vi "WriteData (Array of STR).vi"(6 "value index (0)":u64, 7 "Array of STR":string[](array[string]), 8 "error in (no error)":errorcluster, 9 "channel index (0)":u32, 10 "operation (0: create)":T2(ring)=enum."Create", 11 "Excel refnum":T1) -> (0 "error out":errorcluster, 3 "Excel refnum out":T1)   [LabVIEW 2020, in "NI_ExcelFile.lvlib"]
uses:
  <vilib>/express/express shared/NI_ExcelFile/NI_ExcelFile.lvlib
  <vilib>/express/express shared/NI_ExcelFile/Ctrls/ExcelRefnum.ctl
  <vilib>/express/express shared/NI_ExcelFile/Ctrls/MainData.ctl
  <vilib>/express/express shared/NI_ExcelFile/Ctrls/StreamMode.ctl
  <vilib>/express/express shared/NI_ExcelFile/Ctrls/TimeColumnMode.ctl
  <vilib>/express/express shared/NI_ExcelFile/Ctrls/FileAttribute.ctl
  <vilib>/express/express shared/NI_ExcelFile/Ctrls/Columns.ctl
  <vilib>/express/express shared/NI_ExcelFile/Ctrls/ColumnInfo.ctl
  <vilib>/express/express shared/NI_ExcelFile/Ctrls/DataType.ctl
  <vilib>/express/express shared/NI_ExcelFile/Ctrls/wd_recordInfo.ctl
  <vilib>/express/express shared/NI_ExcelFile/Ctrls/disk_TemplateFile.ctl
  <vilib>/express/express shared/NI_ExcelFile/Ctrls/meta_file.ctl
  <vilib>/express/express shared/NI_ExcelFile/Ctrls/meta_Block.ctl
  <vilib>/express/express shared/NI_ExcelFile/Ctrls/meta_BlockType.ctl
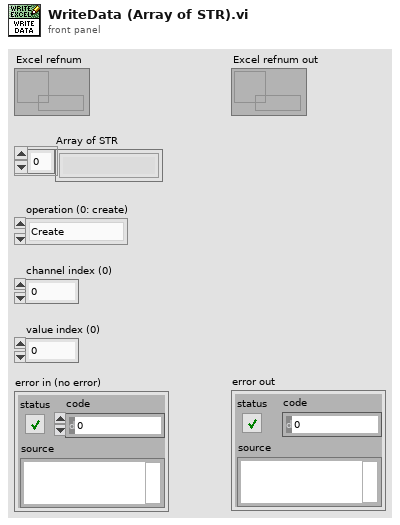
[diagram p1: front panel]
types:
  T1 = typedef "NI_ExcelFile.lvlib/ExcelRefnum.ctl" = refnum<data-value>
  T2 = enum16{"Append values", "Create", "Replace values at index", "Replace all values"}
  T3 = typedef "NI_ExcelFile.lvlib/DataType.ctl" = enum16{"DDT", "WFM", "Array of STR", "Array of DBL", "Array of I8", "Array of I16", "Array of I32", "Array of I64", "Array of SGL", "Array of U8", "Array of U16", "Array of U32", "Array of U64", "Array of Time"}
  T4 = typedef "NI_ExcelFile.lvlib/MainData.ctl" = cluster{"TargetFile":path, "StreamMode":T5, "Append?":bool, "ChunkSize":u64, "TimeColumnMode":T6, "TimestampFormat":string, "AbsoluteTime?":bool, "FileAttribute ":T7, "Column":T8, "FileRef":refnum<k1>, "MemoryRef":refnum<data-value>[], "RecordInfo":T10[], " ChannelPreviousInfo":u32[], "ChannelFirstRecord":u32[], "PredefinedFormattedValueLength":i64, "DiskTemplate":T11}
  T5 = typedef "NI_ExcelFile.lvlib/StreamMode.ctl" = enum16{"File", "Memory"}
  T6 = typedef "NI_ExcelFile.lvlib/TimeColumnMode.ctl" = enum16{"Empty", "OnePerCh", "One"}
  T7 = typedef "NI_ExcelFile.lvlib/FileAttribute.ctl" = cluster{"Creator":string, "Title":string, "SheetName":string}
  T8 = typedef "NI_ExcelFile.lvlib/Columns.ctl" = T9[]
  T9 = typedef "NI_ExcelFile.lvlib/ColumnInfo.ctl" = cluster{"Header":string, "Format":string, "DataType":T3, "Length":u64}
  T10 = typedef "NI_ExcelFile.lvlib/wd_recordInfo.ctl" = cluster{"ChannelIndex":u32, "StartIndex":u64, "Length":u64, "Previous":i32, "Next":i32}
  T11 = typedef "NI_ExcelFile.lvlib/disk_TemplateFile.ctl" = cluster{"XMLRef":refnum<file>[], "ZipPath":path, "MetaFile":T12, "TempFolder":path}
  T12 = typedef "NI_ExcelFile.lvlib/meta_file.ctl" = cluster{"Ref":refnum<file>, "NextRow":i32, "NextPosition":i64, "Block":T13[]}
  T13 = typedef "NI_ExcelFile.lvlib/meta_Block.ctl" = cluster{"Version":u16, "Type":T14, "Length":i32, "Data":string}
  T14 = typedef "NI_ExcelFile.lvlib/meta_BlockType.ctl" = enum16{"NITag", "File", "Column"}
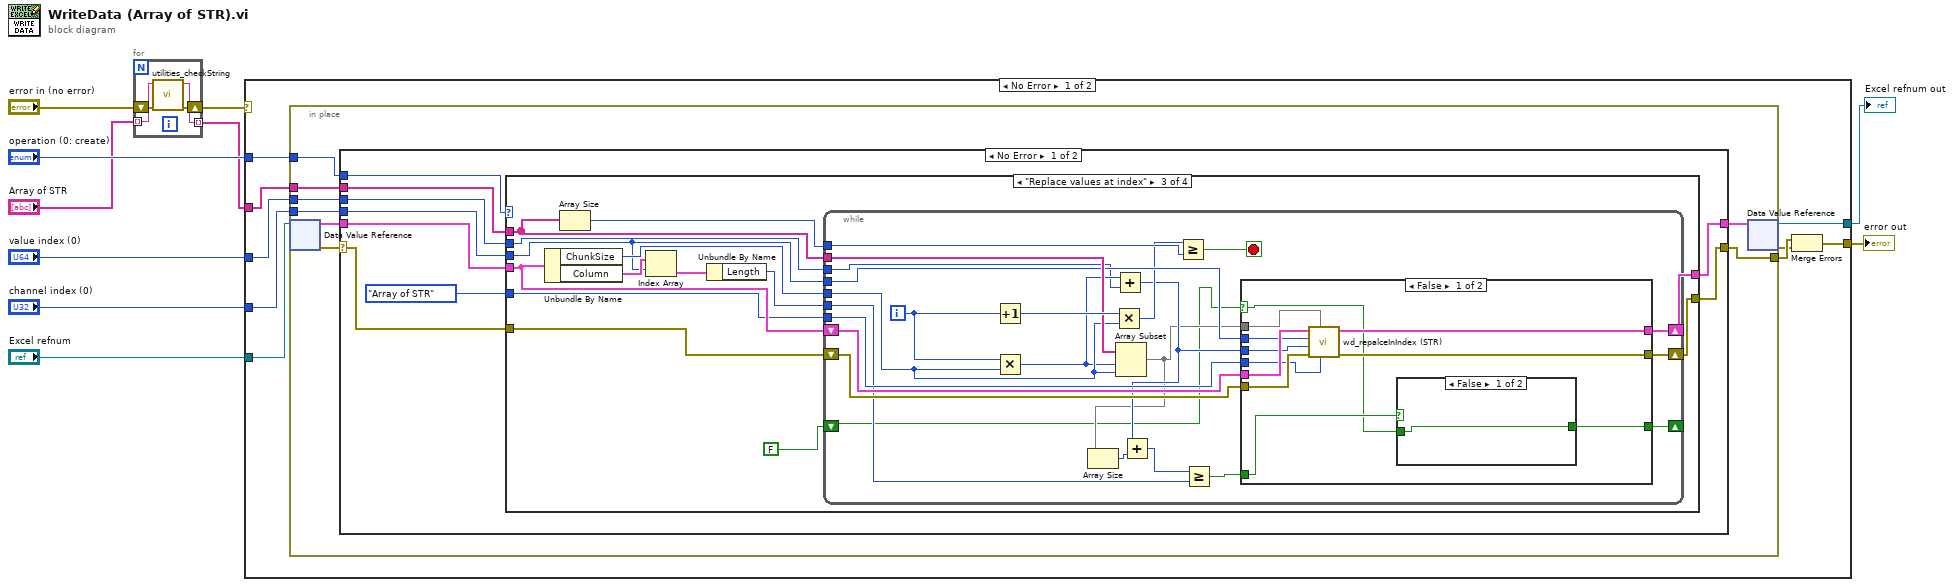
[diagram p0: block diagram]
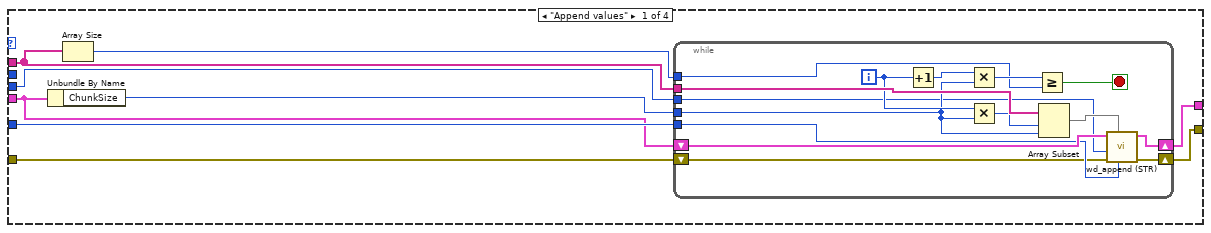
[diagram p2: hidden frame]
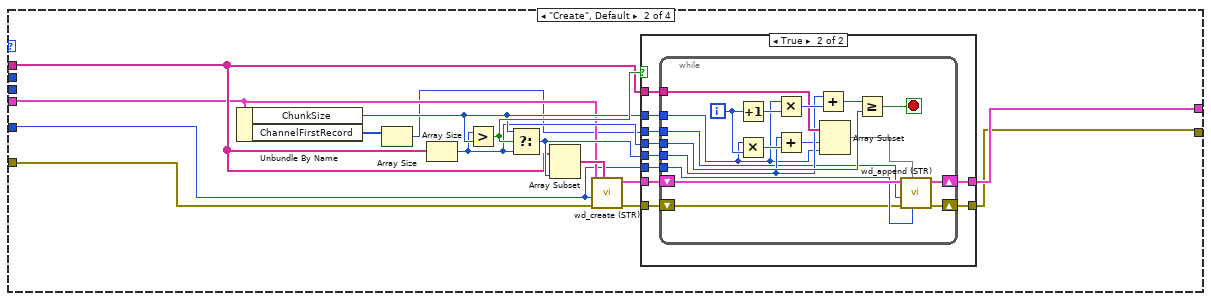
[diagram p3: hidden frame]
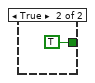
[diagram p5: hidden frame]
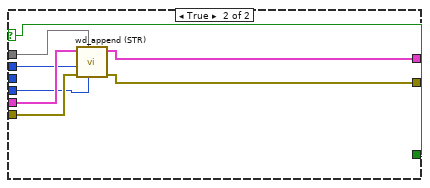
[diagram p6: hidden frame]
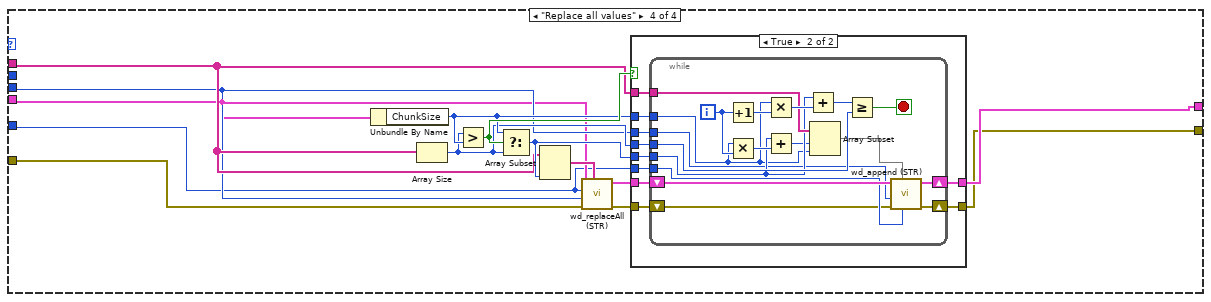
[diagram p7: hidden frame]
diagram:
  n1 = for {
    shift-right: [w13] -> w3
    shift-left: "error in (no error)" -> [w14]
    tunnel: [w12] -> w1 mode=indexing
    tunnel: "Array of STR" -> [w11] mode=indexing
    n2 = call <vilib>:"utilities_checkString.vi"("error in (no error)"=w14, "String"=w11) -> ("error out"=w13:errorcluster, "String out"=w12:string)  [unwired: 8 in]
  }
  n3 = case shown="No Error" w3 {
    selector: w3 -> [_ w215]
    tunnel: w1 -> [w20 _]
    tunnel: [w15 w215] -> w5
    tunnel: "Excel refnum" -> [w23 w214]
    tunnel: [w22 w214] -> w6
    tunnel: "operation (0: create)" -> [w21 _]
    tunnel: "channel index (0)" -> [w19 _]
    tunnel: "value index (0)" -> [w18 _]
    frame No Error {
      n4 = in-place {
        in-place-border: w21 -> [w29]
        in-place-border: w20 -> [w28]
        in-place-border: w19 -> [w27]
        in-place-border: [w26] -> w17
        in-place-border: w18 -> [w25]
        n5 = in-place-dvr #1(w23) -> (w31:T4, w24:errorcluster)
        n6 = case shown="No Error" w24 {
          selector: w24 -> [w32 w212]
          tunnel: w31 -> [w40 w213]
          tunnel: [w39 w213] -> w30
          tunnel: w29 -> [w38 _]
          tunnel: w28 -> [w37 _]
          tunnel: w27 -> [w36 _]
          tunnel: [w35 w212] -> w26
          tunnel: w25 -> [w34 _]
          frame No Error {
            n7 = case shown="\"Replace values at index\"" w38 {
              tunnel: w40 -> [w45 w71 w120 w172]
              tunnel: [w42 w66 w117 w169] -> w39
              tunnel: w37 -> [w48 w72 w121 w174]
              tunnel: w36 -> [w43 _ w114 w173]
              tunnel: w32 -> [w46 w69 w111 w170]
              tunnel: [w41 w65 w116 w168] -> w35
              tunnel: w34 -> [_ _ w118 _]
              tunnel: DataType."Array of STR" ("new element/subarray") -> [w47 w70 w119 w171]
              frame "Append values" {
                n8 = Unbundle By Name(w45) -> ("ChunkSize"=w44:u64)
                n9 = Array Size(array=w48) -> (size(s)=w49:i32)
                n10 = while {
                  tunnel: w44 -> [w54]
                  tunnel: w49 -> [w62]
                  tunnel: w47 -> [w59]
                  tunnel: w48 -> [w57]
                  shift-right: [w51] -> w42
                  shift-left: w45 -> [w60]
                  shift-right: [w52] -> w41
                  shift-left: w46 -> [w58]
                  tunnel: w43 -> [w50]
                  i -> [w56]
                  stop <- w61 stop-if-true
                  n11 = Increment(x=w56) -> (x+1=w64:i32)
                  n12 = Multiply(x=w64, y=w54) -> (x*y=w63:u64)
                  n13 = Multiply(x=w56, y=w54) -> (x*y=w55:u64)
                  n14 = Greater Or Equal?(x=w63, y=w62) -> (x >= y?=w61:bool)
                  n15 = Array Subset(array=w57, index=w55, length=w54) -> (w53:string[])
                  n16 = call <vilib>:"wd_append (STR).vi"("data type"=w59, "data"=w53, "error in (no error)"=w58, "channel index"=w50, "meta in"=w60) -> ("error out"=w52:errorcluster, "meta out"=w51:T4)  [unwired: 5 in]
                }
              }
              frame "Create", Default {
                n17 = Unbundle By Name(w71) -> ("ChunkSize"=w75:u64, "ChannelFirstRecord"=w68:u32[])
                n18 = Array Size(array=w68) -> (size(s)=w67:i32)
                n19 = Array Size(array=w72) -> (size(s)=w73:i32)
                n20 = Greater?(x=w73, y=w75) -> (0:w78:bool)
                n21 = Select(t=w75, s=w78, f=w73) -> (s? t:f=w74:u64)
                n22 = Array Subset(array=w72, length=w74) -> (w79:string[])  [unwired: 1 in]
                n23 = call <vilib>:"wd_create (STR).vi"("data"=w79, "error in (no error)"=w69, "data type"=w70, "meta in"=w71) -> ("error out"=w76:errorcluster, "meta out"=w77:T4)  [unwired: 6 in]
                n24 = case shown="True" w78 {
                  tunnel: [w81 w83] -> w66
                  tunnel: w77 -> [w81 w87]
                  tunnel: [w80 w82] -> w65
                  tunnel: w76 -> [w80 w84]
                  tunnel: w75 -> [_ w91]
                  tunnel: w74 -> [_ w90]
                  tunnel: w73 -> [_ w89]
                  tunnel: w72 -> [_ w88]
                  tunnel: w67 -> [_ w86]
                  tunnel: w70 -> [_ w85]
                  frame False {
                  }
                  frame True {
                    n25 = while {
                      tunnel: w91 -> [w99]
                      tunnel: w90 -> [w101]
                      tunnel: w89 -> [w106]
                      tunnel: w88 -> [w104]
                      shift-right: [w96] -> w83
                      shift-left: w87 -> [w97]
                      tunnel: w86 -> [w95]
                      tunnel: w85 -> [w94]
                      shift-right: [w92] -> w82
                      shift-left: w84 -> [w93]
                      i -> [w103]
                      stop <- w105 stop-if-true
                      n26 = Increment(x=w103) -> (x+1=w109:i32)
                      n27 = Multiply(x=w99, y=w103) -> (x*y=w102:u64)
                      n28 = Multiply(x=w99, y=w109) -> (x*y=w108:u64)
                      n29 = Add(x=w101, y=w102) -> (x+y=w100:u64)
                      n30 = Add(x=w101, y=w108) -> (x+y=w107:u64)
                      n31 = Array Subset(array=w104, index=w100, length=w99) -> (w98:string[])
                      n32 = Greater Or Equal?(x=w107, y=w106) -> (x >= y?=w105:bool)
                      n33 = call <vilib>:"wd_append (STR).vi"("data type"=w94, "data"=w98, "error in (no error)"=w93, "channel index"=w95, "meta in"=w97) -> ("error out"=w92:errorcluster, "meta out"=w96:T4)  [unwired: 5 in]
                    }
                  }
                }
              }
              frame "Replace values at index" {
                n34 = Unbundle By Name(w120) -> ("ChunkSize"=w122:u64, "Column"=w115:T8)
                n35 = Array Size(array=w121) -> (size(s)=w123:i32)
                n36 = Index Array(array=w115, index=w114) -> (element=w113:T9)
                n37 = Unbundle By Name(w113) -> ("Length"=w112:u64)
                n38 = while {
                  tunnel: w122 -> [w141]
                  tunnel: w123 -> [w145]
                  tunnel: w119 -> [w137]
                  tunnel: w121 -> [w143]
                  shift-right: [w136] -> w117
                  shift-left: w120 -> [w139]
                  shift-right: [w135] -> w116
                  shift-left: w111 -> [w138]
                  tunnel: w114 -> [w140]
                  tunnel: w118 -> [w132]
                  tunnel: w112 -> [w130]
                  shift-right: [w124] -> _
                  shift-left: FALSE ("Replace or append?") -> [w125]
                  i -> [w142]
                  stop <- w144 stop-if-true
                  n39 = Increment(x=w142) -> (x+1=w146:i32)
                  n40 = Multiply(x=w142, y=w141) -> (x*y=w134:u64)
                  n41 = Multiply(x=w146, y=w141) -> (x*y=w133:u64)
                  n42 = Add(x=w134, y=w132) -> (x+y=w128:u64)
                  n43 = Array Subset(array=w143, index=w134, length=w141) -> (w126:string[])
                  n44 = Array Size(array=w126) -> (size(s)=w127:i32)
                  n45 = Add(x=w128, y=w127) -> (x+y=w131:u64)
                  n46 = Greater Or Equal?(x=w133, y=w145) -> (x >= y?=w144:bool)
                  n47 = Greater Or Equal?(x=w131, y=w130) -> (x >= y?=w129:bool)
                  n48 = case shown="False" w125 {
                    selector: w125 -> [w148 w160]
                    tunnel: w140 -> [w150 w165]
                    tunnel: w139 -> [w157 w166]
                    tunnel: w126 -> [w156 w167]
                    tunnel: w138 -> [w155 w164]
                    tunnel: w128 -> [w152 _]
                    tunnel: w137 -> [w154 w163]
                    tunnel: [w151 w162] -> w136
                    tunnel: [w153 w161] -> w135
                    tunnel: w129 -> [w149 _]
                    tunnel: [w147 w160] -> w124
                    frame False {
                      n49 = call <vilib>:"wd_repalceInIndex (STR).vi"("data type"=w154, "data"=w156, "error in (no error)"=w155, "value index"=w152, "channel index"=w150, "meta in"=w157) -> ("error out"=w153:errorcluster, "meta out"=w151:T4)  [unwired: 4 in]
                      n50 = case shown="False" w149 {
                        tunnel: w148 -> [w158 _]
                        tunnel: [w158 TRUE] -> w147
                        frame False {
                        }
                        frame True {
                        }
                      }
                    }
                    frame True {
                      n51 = call <vilib>:"wd_append (STR).vi"("data type"=w163, "data"=w167, "error in (no error)"=w164, "channel index"=w165, "meta in"=w166) -> ("error out"=w161:errorcluster, "meta out"=w162:T4)  [unwired: 5 in]
                    }
                  }
                }
              }
              frame "Replace all values" {
                n52 = Unbundle By Name(w172) -> ("ChunkSize"=w177:u64)
                n53 = Array Size(array=w174) -> (size(s)=w175:i32)
                n54 = Greater?(x=w175, y=w177) -> (0:w180:bool)
                n55 = Select(t=w177, s=w180, f=w175) -> (s? t:f=w176:u64)
                n56 = Array Subset(array=w174, length=w176) -> (w181:string[])  [unwired: 1 in]
                n57 = call <vilib>:"wd_replaceAll (STR).vi"("data"=w181, "error in (no error)"=w170, "channel index"=w173, "data type"=w171, "meta in"=w172) -> ("error out"=w178:errorcluster, "meta out"=w179:T4)  [unwired: 5 in]
                n58 = case shown="True" w180 {
                  tunnel: [w183 w185] -> w169
                  tunnel: w179 -> [w183 w189]
                  tunnel: [w182 w184] -> w168
                  tunnel: w178 -> [w182 w186]
                  tunnel: w177 -> [_ w193]
                  tunnel: w176 -> [_ w192]
                  tunnel: w175 -> [_ w191]
                  tunnel: w174 -> [_ w190]
                  tunnel: w173 -> [_ w188]
                  tunnel: w171 -> [_ w187]
                  frame False {
                  }
                  frame True {
                    n59 = while {
                      tunnel: w193 -> [w201]
                      tunnel: w192 -> [w203]
                      tunnel: w191 -> [w208]
                      tunnel: w190 -> [w206]
                      shift-right: [w198] -> w185
                      shift-left: w189 -> [w199]
                      tunnel: w188 -> [w197]
                      tunnel: w187 -> [w196]
                      shift-right: [w194] -> w184
                      shift-left: w186 -> [w195]
                      i -> [w205]
                      stop <- w207 stop-if-true
                      n60 = Increment(x=w205) -> (x+1=w211:i32)
                      n61 = Multiply(x=w201, y=w205) -> (x*y=w204:u64)
                      n62 = Multiply(x=w201, y=w211) -> (x*y=w210:u64)
                      n63 = Add(x=w203, y=w204) -> (x+y=w202:u64)
                      n64 = Add(x=w203, y=w210) -> (x+y=w209:u64)
                      n65 = Array Subset(array=w206, index=w202, length=w201) -> (w200:string[])
                      n66 = Greater Or Equal?(x=w209, y=w208) -> (x >= y?=w207:bool)
                      n67 = call <vilib>:"wd_append (STR).vi"("data type"=w196, "data"=w200, "error in (no error)"=w195, "channel index"=w197, "meta in"=w199) -> ("error out"=w194:errorcluster, "meta out"=w198:T4)  [unwired: 5 in]
                    }
                  }
                }
              }
            }
          }
          frame Error {
          }
        }
        n68 = in-place-dvr #1(w30) -> (w22:T1, w16:errorcluster)
      }
      n69 = Merge Errors(w17, w16) -> (w15:errorcluster)
    }
    frame Error {
    }
  }
  "Excel refnum out" <- w6
  "error out" <- w5
